vi "VCI_CAN_OBJ_To_U8Arr.vi"(1 "VCI_CAN_BUF_T":T1) -> (0 "U8 Arr":u8[](array[numeric]))   [LabVIEW 2011]
uses:
  _USB_CAN_SEND_BUFF_UNIT_.ctl
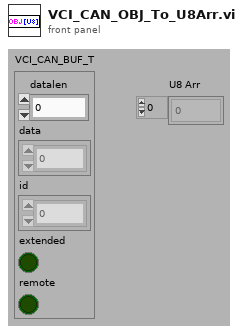
[diagram p1: front panel]
types:
  T1 = typedef "_USB_CAN_SEND_BUFF_UNIT_.ctl" = cluster{"datalen":u8, "data":u8[], "id":u8[], "extended":bool, "remote":bool}
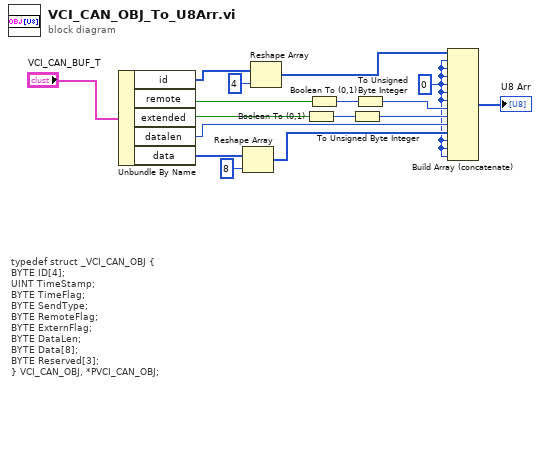
[diagram p0: block diagram]
diagram:
  w2 = u8 0 ("元素")
  # "typedef struct _VCI_CAN_OBJ { \nBYTE ID[4];\nUINT TimeStamp; \nBYTE TimeFlag;\nBYTE SendType; \nBYTE RemoteFlag; \nBYTE ExternFlag; \nBYTE DataLen; \nBYTE Data[8]; \nBYTE Reserved[3];\n} VCI_CAN_OBJ, *PVCI_CAN_OBJ;"
  n1 = Unbundle By Name("VCI_CAN_BUF_T") -> ("id"=w5:u8[], "remote"=w15:bool, "extended"=w11:bool, "datalen"=w9:u8, "data"=w8:u8[])
  n2 = Reshape Array(w8, 8 ("维数大小")) -> (w6:u8[])
  n3 = Reshape Array(w5, 4 ("维数大小")) -> (w3:u8[])
  n4 = Boolean To (0,1)(Boolean=w11) -> (0, 1=w12:i16)
  n5 = Boolean To (0,1)(Boolean=w15) -> (0, 1=w14:i16)
  n6 = To Unsigned Byte Integer(number=w12) -> (unsigned 8bit integer=w10:u8)
  n7 = To Unsigned Byte Integer(number=w14) -> (unsigned 8bit integer=w13:u8)
  n8 = Build Array (concatenate)(w3, w2, w2, w2, w2, w2, w2, w13, w10, w9, w6, w2, w2, w2) -> (→"U8 Arr":u8[])
